vi "trackGlobVar.vi"() -> ()   [LabVIEW 2014]
uses:
  Controls/heinzingerSelect.ctl
panel:
  in  "VoltOrScaler?":bool
  in  "waitAfterReset(25nsTicks)":u16 caption="waitForDmm(25nsTicks)"
  in  "waitForKepco(25nsTicks)":u16
  in  "heinzingerControl":T1
  out "invertScan":bool
  in  "nOfScans":i32
  in  "nOfSteps":i32
  in  "start":i32
  in  "stepSize":i32
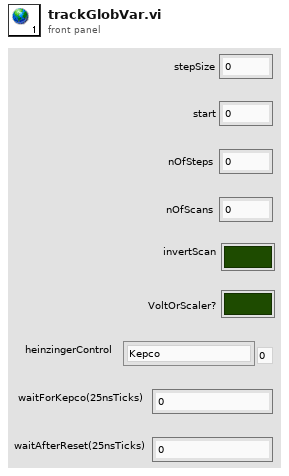
[diagram p1: front panel]
types:
  T1 = typedef "heinzingerSelect.ctl" = enum8{"Kepco", "Heinzinger0", "Heinzinger1", "Heinzinger2", "loading"}
diagram:
